vi "PS_Cycling.vi"(0 "Keithley 2400 PULL-UP Actuator PS":refnum<visa-resource-name>="GPIB0::3::INSTR", 1 "Current Limit Pull-Up(A)":dbl=0.1, 2 "Cycling Setup":bool, 3 "Current Limit Pull-DN (A)":dbl=0.1, 5 "Keithley 2400 PULL-DN Actuator PS":refnum<visa-resource-name>="GPIB0::3::INSTR", 7 "Cycling Cluster":T1, 11 "Error In":errorcluster, 14 "Index":i32) -> (15 "error out":errorcluster)   [LabVIEW 2017]
uses:
  Controls/Cycling_Cluster.ctl
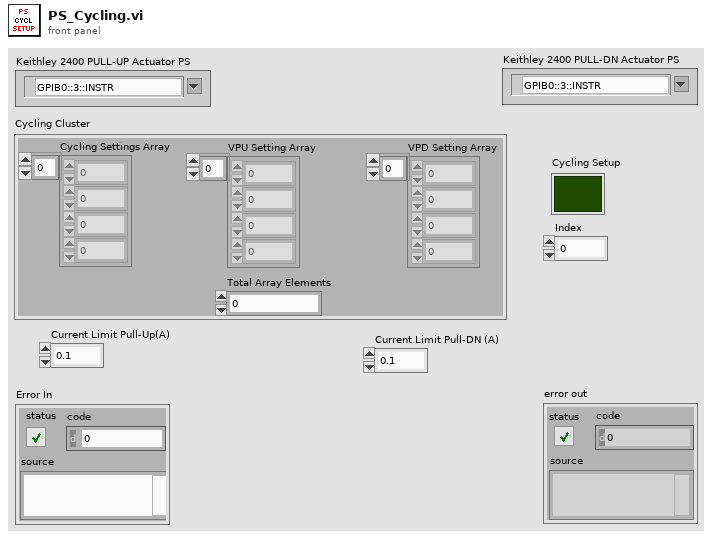
[diagram p1: front panel]
types:
  T1 = typedef "Cycling_Cluster.ctl" = cluster{"Cycling Settings Array":i64[], "VPU Setting Array":i64[], "VPD Setting Array":i64[], "Total Array Elements":i32}
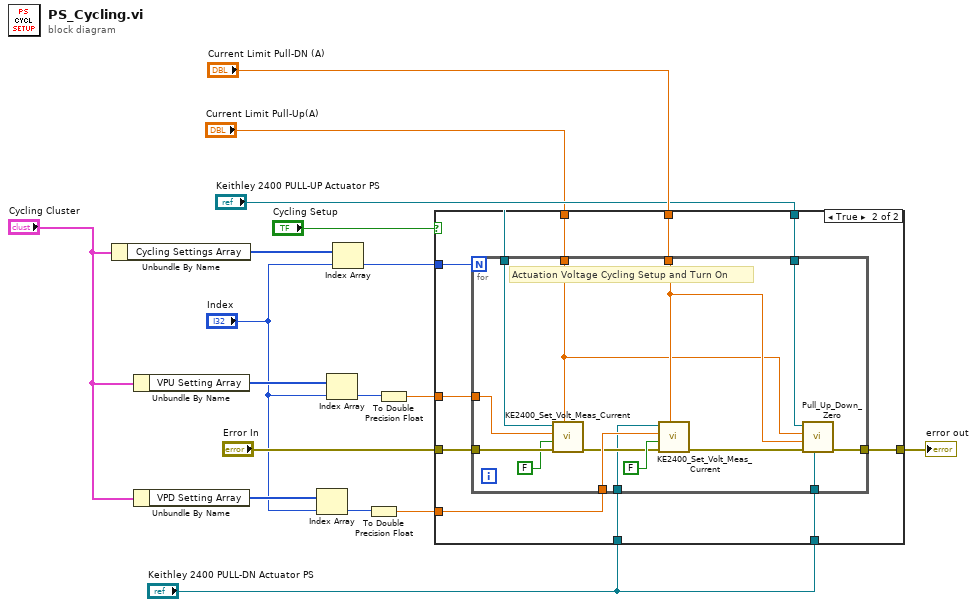
[diagram p0: block diagram]
diagram:
  n1 = Unbundle By Name("Cycling Cluster") -> ("Cycling Settings Array"=w11:i64[])
  n2 = Unbundle By Name("Cycling Cluster") -> ("VPU Setting Array"=w8:i64[])
  n3 = Unbundle By Name("Cycling Cluster") -> ("VPD Setting Array"=w3:i64[])
  n4 = Index Array(array=w3, index="Index") -> (element=w4:i64)
  n5 = Index Array(array=w8, index="Index") -> (element=w7:i64)
  n6 = Index Array(array=w11, index="Index") -> (element=w10:i64)
  n7 = To Double Precision Float(number=w4) -> (double precision float=w1:dbl)
  n8 = To Double Precision Float(number=w7) -> (double precision float=w6:dbl)
  n9 = case shown="True" "Cycling Setup" {
    tunnel: "Error In" -> [w18 w28]
    tunnel: w1 -> [_ w27]
    tunnel: "Current Limit Pull-DN (A)" -> [_ w26]
    tunnel: [w18 w25] -> w15
    tunnel: "Keithley 2400 PULL-DN Actuator PS" -> [_ w24]
    tunnel: "Keithley 2400 PULL-UP Actuator PS" -> [_ w23]
    tunnel: w10 -> [_ w22]
    tunnel: "Keithley 2400 PULL-DN Actuator PS" -> [_ w21]
    tunnel: "Current Limit Pull-Up(A)" -> [_ w20]
    tunnel: w6 -> [_ w19]
    frame False {
    }
    frame True {
      n10 = for {
        N: w22 -> [_]
        tunnel: w27 -> [w41]
        tunnel: w23 -> [w40]
        tunnel: w24 -> [w39]
        tunnel: w26 -> [w38]
        tunnel: w28 -> [w42]
        tunnel: [w37] -> w25
        tunnel: w21 -> [w32]
        tunnel: w23 -> [w31]
        tunnel: w20 -> [w30]
        tunnel: w19 -> [w29]
        # "Actuation Voltage Cycling Setup and Turn On"
        n11 = call "KE2400_Set_Volt_Meas_Current.vi"("Compliance  Level (0.1)"=w30, "error in (no error)"=w42, "Enable Remote Sensing (T: Enable)"=FALSE, "Output Level (0)"=w29, "VISA resource name"=w31) -> ("error out"=w34:errorcluster)  [unwired: 4 in, 2 out]
        n12 = call "KE2400_Set_Volt_Meas_Current.vi"("Compliance  Level (0.1)"=w38, "error in (no error)"=w34, "Enable Remote Sensing (T: Enable)"=FALSE, "Output Level (0)"=w41, "VISA resource name"=w32) -> ("error out"=w33:errorcluster)  [unwired: 4 in, 2 out]
        n13 = call "Pull_Up_Down_Zero.vi"("Keithley 2400 Actuator Pull-DN PS"=w39, "error in (no error)"=w33, "Current Limit Pull-DN (A)"=w38, "Current Limit Pull-Up(A)"=w30, "Keithley 2400 Actuator Pull-Up PS"=w40) -> ("error out"=w37:errorcluster)  [unwired: 6 in]
      }
    }
  }
  "error out" <- w15
